vi "Find By Both.vi"(11 "Both":string) -> (2 "Found?":bool, 3 "Team Data":T1)   [LabVIEW 2013]
uses:
  Team Data.ctl
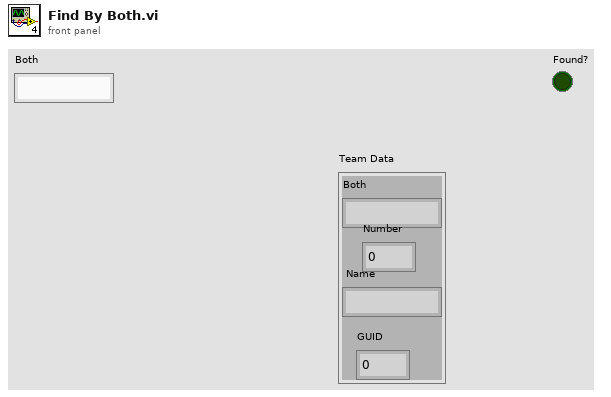
[diagram p1: front panel]
types:
  T1 = typedef "Team Data.ctl" = cluster{"Both":string, "Name":string, "GUID":u16, "Number":u16}
  T2 = enum16{"Get Teams", "Add Team", "Modify Team", "Clear All Teams", "Force Add Team", "Delete Team"}
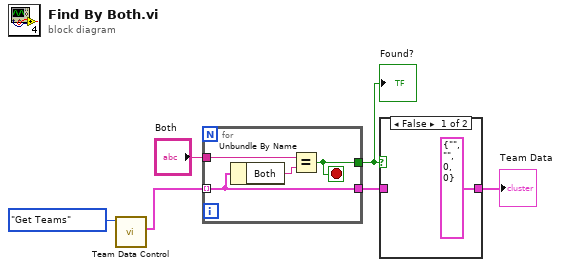
[diagram p0: block diagram]
diagram:
  n1 = call "Team Data Control.vi"("Mode"=T2."Get Teams") -> ("Team Array Out"=w1:T1[])  [unwired: 10 in]
  n2 = for {
    tunnel: w1 -> [w8] mode=indexing
    tunnel: [w9] -> w6
    tunnel: [w8] -> w5
    tunnel: "Both" -> [w7]
    stop <- w9 stop-if-true
    n3 = Unbundle By Name(w8) -> ("Both"=w10:string)
    n4 = Equal?(x=w7, y=w10) -> (x = y?=w9:bool)
  }
  "Found?" <- w6
  n5 = case shown="False" w6 {
    tunnel: [T1 {"Both"="", "Name"="", "GUID"=0, "Number"=0} ("Team Data") w12] -> w4
    tunnel: w5 -> [_ w12]
    frame False {
    }
    frame True {
    }
  }
  "Team Data" <- w4
